vi "AuMT8852B Path Offset Table Entry Delete.vi"(5 "Frequency units (Channel)":enum16{"Channel", "MHz"}(ring), 7 "Frequency (Channel 0)":i32, 8 "error in (no error)":errorcluster, 10 "Table (1)":i32=1, 11 "VISA session":refnum<visa-resource-name>) -> (0 "error out":errorcluster, 2 "error code":i32, 3 "VISA session out":refnum<visa-resource-name>)   [LabVIEW 2017]
doc: "Anritsu MT8852B Bluetooth Tester\n\nDeletes the offset for a particular frequency or channel in the selected path offset table.\n\nINPUTS\nTable - path offset table (1-10) to use.\nFrequency - frequency whose the offset will be deleted.\nFrequency units - whether the frequency is expressed as a channel or a frequency in MHz."
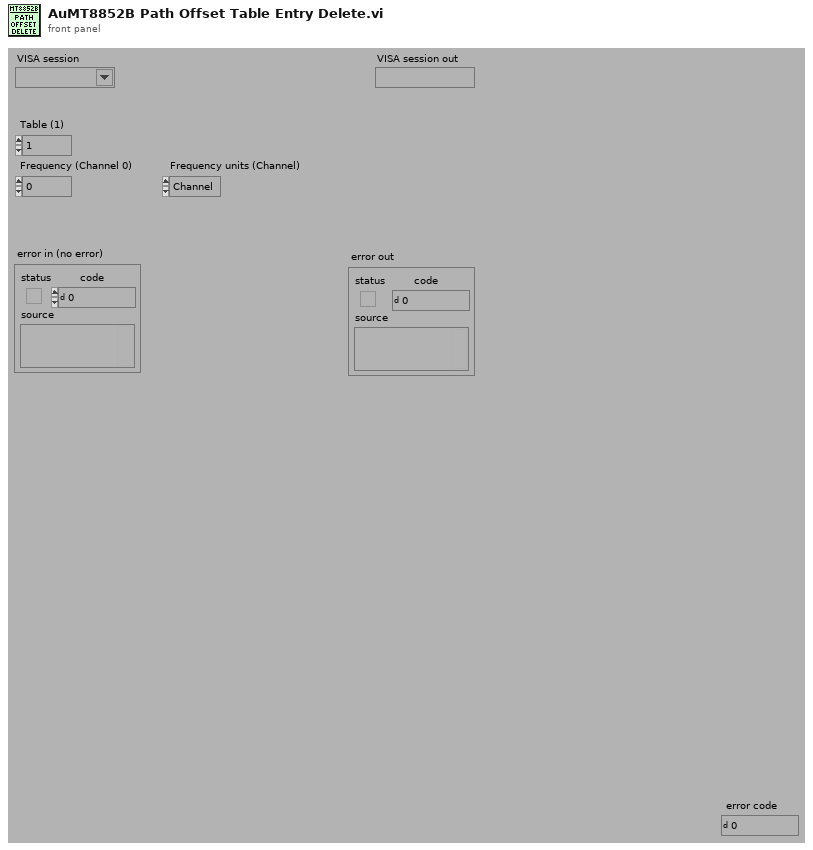
[diagram p1: front panel]
types:
  T1 = enum16{"Simulate", "Range check", "Cache", "Query instrument status"}
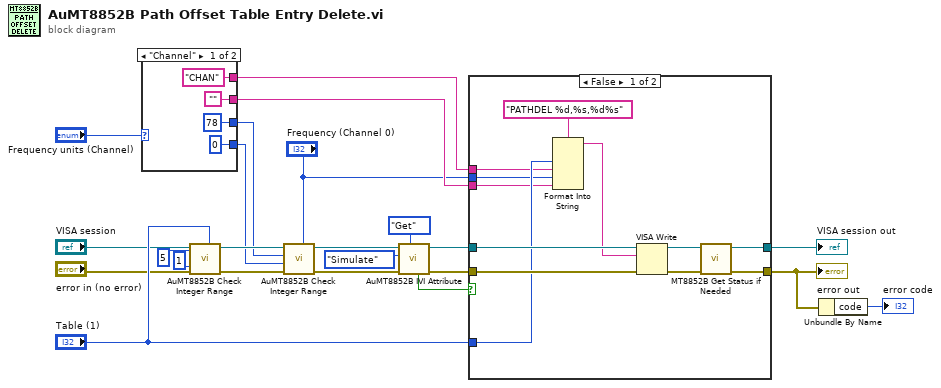
[diagram p0: block diagram]
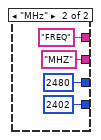
[diagram p2: hidden frame]
diagram:
  n1 = case shown="\"Channel\"" "Frequency units (Channel)" {
    tunnel: [0 2402] -> w9
    tunnel: [78 2480] -> w8
    tunnel: ["" "MHZ"] -> w5
    tunnel: ["CHAN" "FREQ"] -> w3
    frame "Channel" {
    }
    frame "MHz" {
    }
  }
  n2 = call <instrlib>:"AuMT8852B Check Integer Range.vi"("Value (0)"="Table (1)", "error in (no error)"="error in (no error)", "Lower limit (-1)"=1, "Upper limit (1)"=5, "VISA session"="VISA session") -> ("error out"=w12:errorcluster, "VISA session out"=w11:refnum<visa-resource-name>)  [unwired: 5 in]
  n3 = call <instrlib>:"AuMT8852B Check Integer Range.vi"("Value (0)"="Frequency (Channel 0)", "error in (no error)"=w12, "Lower limit (-1)"=w9, "Upper limit (1)"=w8, "VISA session"=w11) -> ("error out"=w2:errorcluster, "VISA session out"=w1:refnum<visa-resource-name>)  [unwired: 5 in]
  n4 = call <instrlib>:"AuMT8852B IVI Attribute.vi"("Set/Get (Set)"=enum16{"Set", "Get"}."Get", "error in (no error)"=w2, "Flag (Simulate)"=T1."Simulate", "VISA session"=w1) -> ("error out"=w21:errorcluster, "VISA session out"=w22:refnum<visa-resource-name>, "Value out"=w18:bool)  [unwired: 5 in]
  n5 = case shown="False" w18 {
    tunnel: [w37 w45] -> w23
    tunnel: [w38 w44] -> w16
    tunnel: w22 -> [w43 w45]
    tunnel: w21 -> [w42 w44]
    tunnel: "Table (1)" -> [w41 _]
    tunnel: w5 -> [w36 _]
    tunnel: "Frequency (Channel 0)" -> [w35 _]
    tunnel: w3 -> [w34 _]
    frame False {
      n6 = Format Into String(format string="PATHDEL %d,%s,%d%s" ("Command ()"), w41, w34, w35, w36) -> (resulting string=w32:string)  [unwired: 2 in, 1 out]
      n7 = VISA Write(VISA resource name=w43, write buffer=w32, error in (no error)=w42) -> (VISA resource name out=w39:refnum<visa-resource-name>, error out=w40:errorcluster)  [unwired: 1 out]
      n8 = call <instrlib>:"MT8852B Get Status if Needed.vi"("error in (no error)"=w40, "VISA session"=w39) -> ("error out"=w38:errorcluster, "VISA session out"=w37:refnum<visa-resource-name>)  [unwired: 8 in]
    }
    frame True {
      (unwired) "" ("Response")
    }
  }
  "error out" <- w16
  "VISA session out" <- w23
  n9 = Unbundle By Name(w16) -> ("code"=→"error code":i32)
